vi "SEA_9811_ARINCdata2word_FPGA.vi"(7 "Reverse label bits":bool, 9 "Data":u32, 10 "SDI":u8, 11 "Label":u8) -> (3 "ARINC word out":T1 format="%032b")   [LabVIEW 2012]
doc: "Calculate ARINC word incl. odd parity from label, SDI and data. Optimized for FPGA usage."
uses:
  Typdefs/ARINC word.ctl
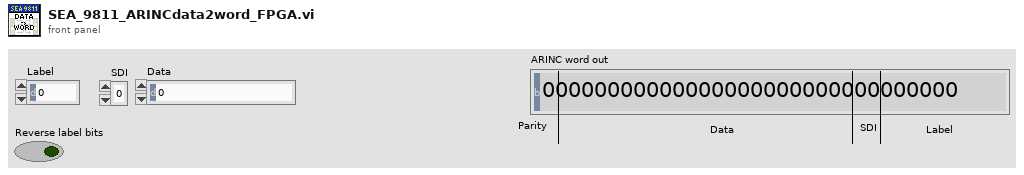
[diagram p1: front panel]
types:
  T1 = typedef "ARINC word.ctl" = u32
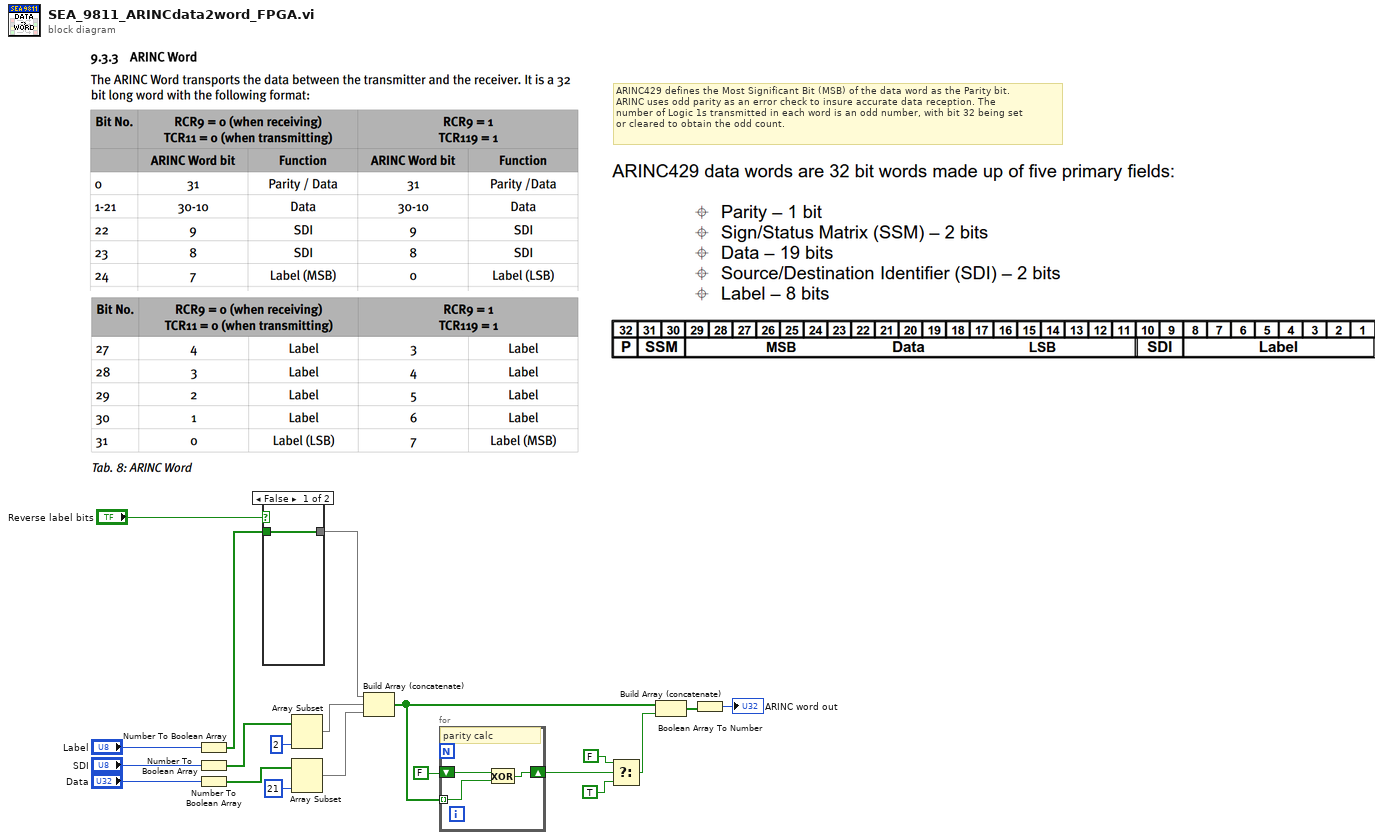
[diagram p0: block diagram]
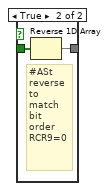
[diagram p2: hidden frame]
diagram:
  # "ARINC429 defines the Most Significant Bit (MSB) of the data word as the Parity bit.\nARINC uses odd parity as an error check to insure accurate data reception. The\nnumber of Logic 1s transmitted in each word is an odd number, with bit 32 being set\nor cleared to obtain the odd count."
  n1 = Number To Boolean Array(number="Label") -> (Boolean array=w12:bool[])
  n2 = Number To Boolean Array(number="SDI") -> (Boolean array=w16:bool[])
  n3 = Number To Boolean Array(number="Data") -> (Boolean array=w19:bool[])
  n4 = case shown="False" "Reverse label bits" {
    tunnel: [w21 w23] -> w13
    tunnel: w12 -> [w21 w22]
    frame False {
    }
    frame True {
      # "#ASt\nreverse\nto \nmatch\nbit\norder\nRCR9=0"
      n5 = Reverse 1D Array(array=w22) -> (reversed array=w23:bool[])
    }
  }
  n6 = Array Subset(array=w16, length=2) -> (w15:bool[])  [unwired: 1 in]
  n7 = Array Subset(array=w19, length=21) -> (w14:bool[])  [unwired: 1 in]
  n8 = Build Array (concatenate)(w13, w15, w14) -> (w9:bool[])
  n9 = for {
    shift-right: [w26] -> w7
    shift-left: FALSE -> [w25]
    tunnel: w9 -> [w24] mode=indexing
    # "parity calc"
    n10 = Exclusive Or(1:w24, 2:w25) -> (0:w26:bool)
  }
  n11 = Select(t=FALSE, s=w7, f=TRUE) -> (s? t:f=w5:bool)
  n12 = Build Array (concatenate)(w9, w5) -> (w8:bool[])
  n13 = Boolean Array To Number(Boolean array=w8) -> (number=→"ARINC word out":u32)
